vi "MK210-301_GenerateErrorDescr.vi"(4 "Error Code":i32=5490, 6 "Driver Name":string="B1_28", 8 "error in":errorcluster, 11 "status byte":u16 format="%b") -> (0 "error out":errorcluster)   [LabVIEW 2018]
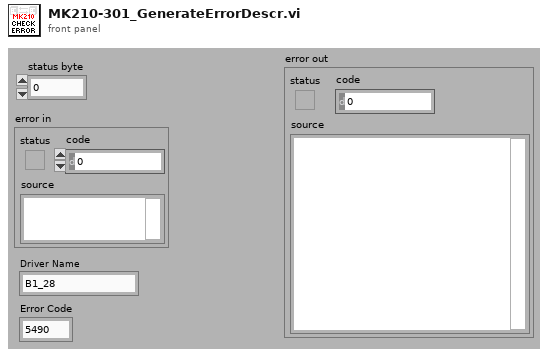
[diagram p1: front panel]
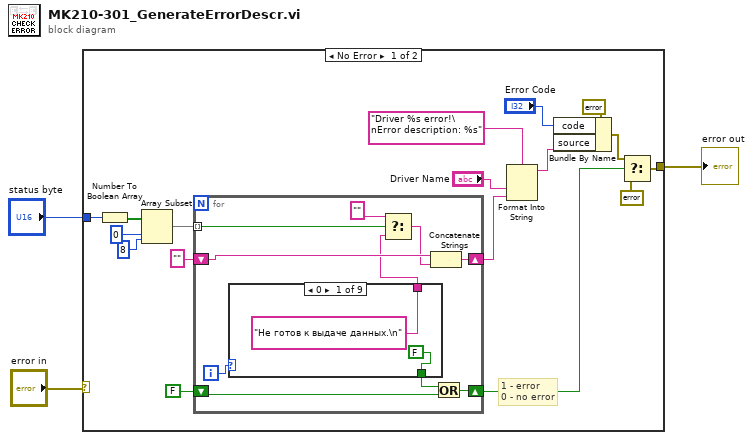
[diagram p0: block diagram]
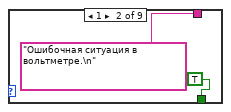
[diagram p2: hidden frame]
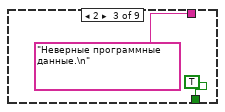
[diagram p3: hidden frame]
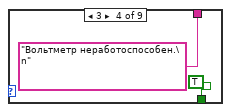
[diagram p4: hidden frame]
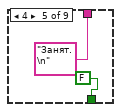
[diagram p5: hidden frame]
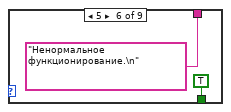
[diagram p6: hidden frame]
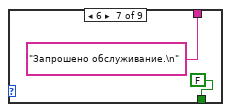
[diagram p7: hidden frame]
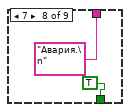
[diagram p8: hidden frame]
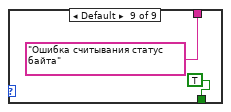
[diagram p9: hidden frame]
diagram:
  n1 = case shown="No Error" "error in" {
    selector: "error in" -> [_ w49]
    tunnel: [w14 w49] -> w2
    tunnel: "status byte" -> [w12 _]
    frame No Error {
      # "1 - error\n0 - no error"
      n2 = Number To Boolean Array(number=w12) -> (Boolean array=w11:bool[])
      n3 = Array Subset(array=w11, index=0, length=8) -> (w8:bool[])
      n4 = for {
        tunnel: w8 -> [w29] mode=indexing
        shift-right: [w27] -> w6
        shift-left: "" ("Driver Name") -> [w28]
        shift-right: [w23] -> w4
        shift-left: FALSE -> [w22]
        i -> [w30]
        n5 = case shown="0" w30 {
          tunnel: ["Не готов к выдаче данных.\n" ("Driver Name") "Ошибочная ситуация в вольтметре.\n" ("Driver Name") "Неверные программные данные.\n" ("Driver Name") "Вольтметр неработоспособен.\n" ("Driver Name") "Занят.\n" ("Driver Name") "Ненормальное функционирование.\n" ("Driver Name") "Запрошено обслуживание.\n" ("Driver Name") "Авария.\n" ("Driver Name") "Ошибка считывания статус байта" ("Driver Name")] -> w25
          tunnel: [FALSE TRUE TRUE TRUE FALSE TRUE FALSE TRUE TRUE] -> w21
          frame 0 {
          }
          frame 1 {
          }
          frame 2 {
          }
          frame 3 {
          }
          frame 4 {
          }
          frame 5 {
          }
          frame 6 {
          }
          frame 7 {
          }
          frame Default {
          }
        }
        n6 = Select(t="" ("Driver Name"), s=w29, f=w25) -> (s? t:f=w24:string)
        n7 = Concatenate Strings(w28, w24) -> (w27:string)
        n8 = Or(x=w21, y=w22) -> (x .or. y?=w23:bool)
      }
      n9 = Format Into String(format string="Driver %s error!\nError description: %s", "Driver Name", w6) -> (resulting string=w18:string)  [unwired: 2 in, 1 out]
      n10 = Bundle By Name(cluster=errorcluster {"status"=TRUE, "code"=0, "source"=""} ("error in"), "code"="Error Code", "source"=w18) -> (w15:errorcluster)
      n11 = Select(t=w15, s=w4, f=errorcluster {"status"=FALSE, "code"=0, "source"=""}) -> (s? t:f=w14:errorcluster)
    }
    frame Error {
    }
  }
  "error out" <- w2
